vi "Update Available COMM List.vi"(8 "error in (no error)":errorcluster, 11 "Controller in":refnum<class "Controller.lvclass">) -> (0 "error out":errorcluster, 3 "Controller out":refnum<class "Controller.lvclass">)   [LabVIEW 2016, in "Controller Actor.lvlib" / "Controller.lvclass"]
uses:
  <userlib>/Common Components/Controller/Controller.lvclass
  <userlib>/Common Components/Controller UI/Update DT event data.ctl
  <userlib>/Common Components/Controller UI/Update DT Cmd.ctl
  <userlib>/Common Components/Controller/Controller.lvclass/Controller.ctl
  <userlib>/Common Components/Hardware/Abstract Hardware/Hardware.lvclass
  <userlib>/Common Components/Controller UI Messages/Update DT Event Msg/Update DT Event Msg.lvclass/Update DT Event Msg.ctl
  <vilib>/ActorFramework/Message Enqueuer/Message Enqueuer.lvclass/Message Enqueuer.ctl
  <vilib>/ActorFramework/Message Enqueuer/Enqueue.vi
  <userlib>/Common Components/Controller UI Messages/Update DT Event Msg/Update DT Event Msg.lvclass
  C:/Program Files (x86)/National Instruments/LabVIEW 2016/vi.lib/ActorFramework/Message/Message.lvclass
  <vilib>/ActorFramework/Message Priority Queue/Priority Enqueue.vi
  <userlib>/Common Components/Controller UI/Controller UI.lvclass
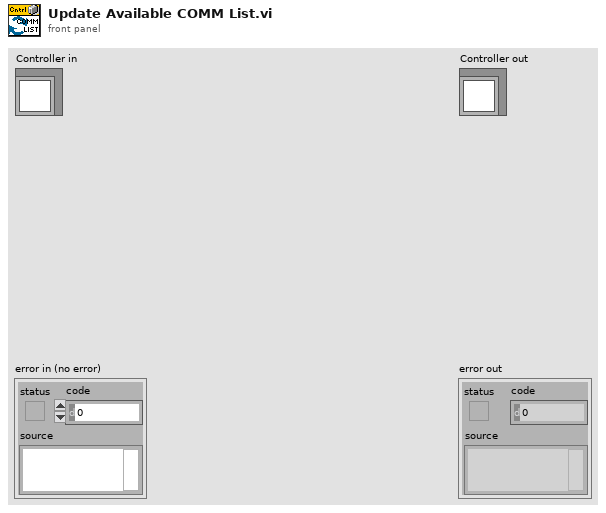
[diagram p1: front panel]
types:
  T1 = typedef "Controller UI.lvlib/Controller UI.lvclass/Update DT event data.ctl" = cluster{"Cmd":T2, "Data Array":variant[]}
  T2 = typedef "Controller UI.lvlib/Controller UI.lvclass/Update DT Cmd.ctl" = enum16{"Update HWtype\\HWplugin array", "Update Checked-out", "Update COMM Status", "Load DevInfo from File", "Save DevInfo to File", "Update COMM Address List"}
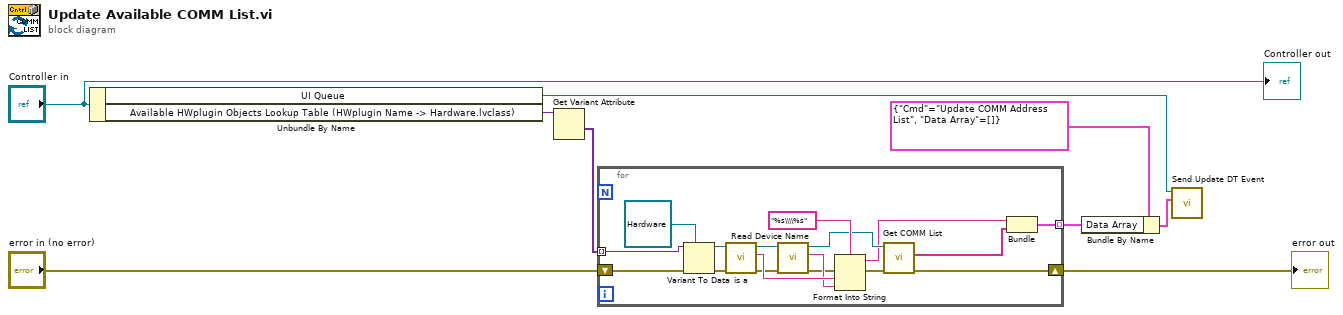
[diagram p0: block diagram]
diagram:
  n1 = Unbundle By Name("Controller in") -> ("UI Queue"=w6:refnum<class "Message Enqueuer.lvclass">, "Available HWplugin Objects Lookup Table (HWplugin Name -> Hardware.lvclass)"=w8:variant)
  n2 = Get Variant Attribute(Variant=w8) -> (values=w7:variant[])  [unwired: 3 in, 3 out]
  n3 = for {
    tunnel: w7 -> [w26] mode=indexing
    tunnel: [w23] -> w4 mode=indexing
    shift-right: [w21] -> w1
    shift-left: "error in (no error)" -> [w22]
    n4 = Variant To Data(error in=w22, type=refnum<class "Hardware.lvclass"> refnum ("Hardware.lvlib:Hardware.lvclass"), Variant=w26) -> (data=w14:refnum<class "Hardware.lvclass">, error out=w13:errorcluster)
    n5 = call-dynamic "is a.vi"("error in (no error)"=w13, "Hardware in"=w14) -> ("error out"=w16:errorcluster, "is a"=w18:string, "Hardware out"=w20:refnum<class "Hardware.lvclass">)  [unwired: 7 in]
    n6 = call <userlib>:"Read Device Name.vi"("error in (no error)"=w16, "Analog in"=w20) -> ("error out"=w15:errorcluster, "Device Name"=w17:string, "Analog out"=w12:refnum<class "Hardware.lvclass">)  [unwired: 7 in]
    n7 = Format Into String(format string="%s\\\\%s", error in=w15, w18, w17) -> (resulting string=w10:string, error out=w11:errorcluster)  [unwired: 1 in]
    n8 = call-dynamic "Get COMM List.vi"("error in (no error)"=w11, "Hardware in"=w12) -> ("error out"=w21:errorcluster, "COMM List"=w24:string[])  [unwired: 7 in, 1 out]
    n9 = Bundle(w10, "COMM List"=w24) -> (w23:cluster{string, "COMM List":string[]})  [unwired: 1 in]
  }
  "error out" <- w1
  n10 = Bundle By Name(cluster=T1 {"Cmd"=enum."Update COMM Address List", "Data Array"=[]} ("event data"), "Data Array"=w4) -> (w5:T1)
  n11 = call <userlib>:"Send Update DT Event.vi"("event data"=w5, "Message Enqueuer"=w6) -> ()  [unwired: 8 in, 2 out]
  "Controller out" <- "Controller in"
